vi "Apply Step Result.vi"(8 "error in (no error)":errorcluster, 9 "ResultStatus":string, 10 "UniqueStepId":string, 11 "Steps Tree In":refnum<vi>) -> (0 "error out":errorcluster, 3 "Steps Tree":refnum<vi>)   [LabVIEW 2020, in "TSnax UI.lvlib" / "SequenceViewPanel.lvclass"]
uses:
  SequenceViewPanel.lvclass
  SequenceViewPanel.lvclass/SequenceViewPanel.ctl
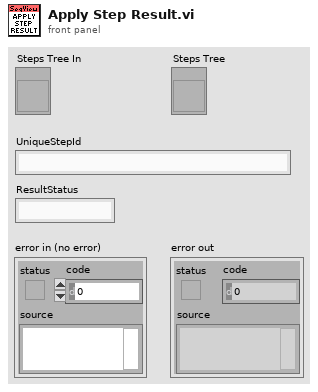
[diagram p1: front panel]
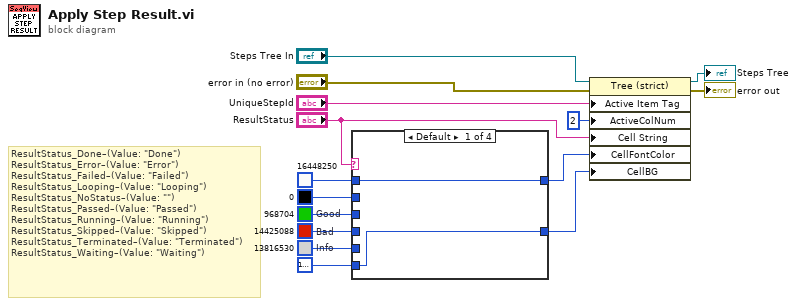
[diagram p0: block diagram]
diagram:
  w11 = u32 968704  # Good
  w12 = u32 14425088  # Bad
  w13 = u32 13816530  # Info
  # "ResultStatus_Done–(Value: \"Done\")\nResultStatus_Error–(Value: \"Error\")\nResultStatus_Failed–(Value: \"Failed\")\nResultStatus_Looping–(Value: \"Looping\")\nResultStatus_NoStatus–(Value: \"\")\nResultStatus_Passed–(Value: \"Passed\")\nResultStatus_Running–(Value: \"Running\")\nResultStatus_Skipped–(Value: \"Skipped\")\nResultStatus_Terminated–(Value: \"Terminated\")\nResultStatus_Waiting–(Value: \"Waiting\")"
  n1 = case shown="Default" "ResultStatus" {
    tunnel: w13 -> [_ _ _ _]
    tunnel: w12 -> [_ _ w21 _]
    tunnel: w11 -> [_ _ _ w22]
    tunnel: u32 0 -> [_ w19 _ _]
    tunnel: u32 16448250 -> [w16 _ w20 w23]
    tunnel: [w17 w18 w21 w22] -> w7
    tunnel: [w16 w19 w20 w23] -> w8
    tunnel: u32 16777216 -> [w17 w18 _ _]
    frame Default {
    }
    frame "" {
    }
    frame "Error", "Failed", "Terminated" {
    }
    frame "Passed" {
    }
  }
  n2 = property class="Tree (strict)"(reference="Steps Tree In", error in="error in (no error)", "Active Item Tag"="UniqueStepId", "ActiveColNum"=2 ("Active Cell:Active Column Number"), "Cell String"="ResultStatus", "CellFontColor"=w8, "CellBG"=w7) -> (reference out=→"Steps Tree":refnum<vi>, error out=→"error out":errorcluster)
